vi "Configure Arbitrary Waveform.vi"(6 "Offset (0.00 V)":dbl, 7 "Frequency (1000 Hz)":dbl=1000.0, 8 "error in (no error)":errorcluster, 9 "Gain (1.0 Vpp)":dbl=1.0, 10 "Arbitrary Waveform Name (\"ARB1\")":string="ARB1", 11 "VISA resource name":refnum<visa-resource-name>) -> (0 "error out":errorcluster, 3 "VISA resource name out":refnum<visa-resource-name>)   [LabVIEW 2015, in "Template - Function Generator.lvlib"]
doc: "Sets the waveform parameters for an arbitrary waveform and make it the active waveform function. This VI should be called after <b>Create Arbitrary Waveform</b> VI."
uses:
  <instrlib>/_Template - Function Generator/Template - Function Generator.lvlib
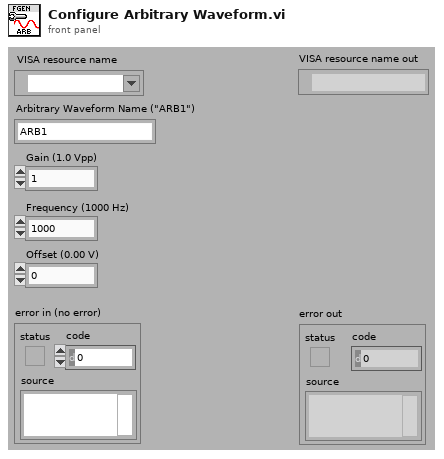
[diagram p1: front panel]
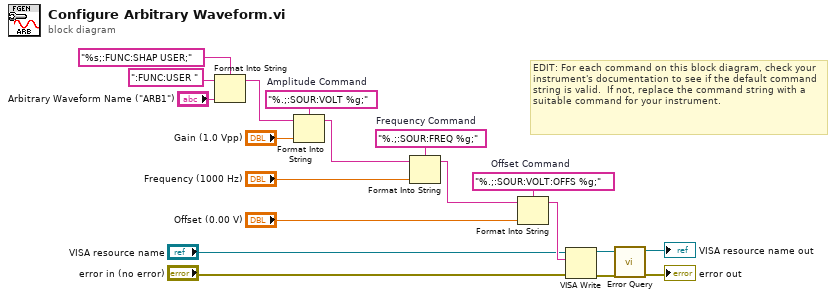
[diagram p0: block diagram]
diagram:
  w3 = "%.;:SOUR:VOLT:OFFS %g;"  # Offset Command
  w19 = "%.;:SOUR:VOLT %g;"  # Amplitude Command
  w4 = "%.;:SOUR:FREQ %g;"  # Frequency Command
  # "EDIT: For each command on this block diagram, check your instrument's documentation to see if the default command string is valid.  If not, replace the command string with a suitable command for your instrument."
  n1 = Format Into String(format string="%s;:FUNC:SHAP USER;", initial string=":FUNC:USER ", "Arbitrary Waveform Name (\"ARB1\")") -> (resulting string=w11:string)  [unwired: 1 in, 1 out]
  n2 = Format Into String(format string=w19, initial string=w11, "Gain (1.0 Vpp)") -> (resulting string=w17:string)  [unwired: 1 in, 1 out]
  n3 = Format Into String(format string=w4, initial string=w17, "Frequency (1000 Hz)") -> (resulting string=w16:string)  [unwired: 1 in, 1 out]
  n4 = Format Into String(format string=w3, initial string=w16, "Offset (0.00 V)") -> (resulting string=w15:string)  [unwired: 1 in, 1 out]
  n5 = VISA Write(VISA resource name="VISA resource name", write buffer=w15, error in (no error)="error in (no error)") -> (VISA resource name out=w10:refnum<visa-resource-name>, error out=w9:errorcluster)  [unwired: 1 out]
  n6 = call <instrlib>:"Error Query.vi"("error in (no error)"=w9, "VISA resource name"=w10) -> ("error out"=→"error out":errorcluster, "VISA resource name out"=→"VISA resource name out":refnum<visa-resource-name>)  [unwired: 6 in, 2 out]
